vi "GenerateTdms.vi"   [LabVIEW 2011]
uses:
  <vilib>/Analysis/NI_AALBase.lvlib
types:
  T1 = enum16{"open", "open or create", "create or replace", "create", "open (read-only)"}
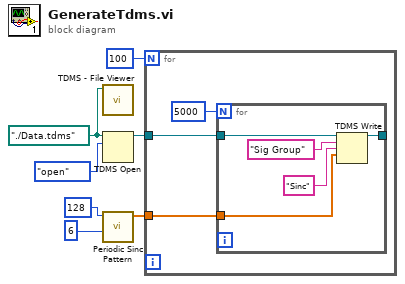
[diagram p0: block diagram]
diagram:
  w5 = path "./Data.tdms" ("文件路径")
  n1 = call <vilib>:"TDMS - File Viewer.vi"("file path"=w5) -> ()  [unwired: 5 in, 2 out]
  n2 = TDMS Open(10:T1."open" ("操作(0:open)"), 11:w5) -> (3:w6:refnum<k34>)  [unwired: 4 in, 1 out]
  n3 = call <vilib>:"Periodic Sinc Pattern.vi"("order"=6, "samples"=128) -> ("Periodic Sinc Pattern"=w2:dbl[])  [unwired: 8 in, 1 out]
  n4 = for {
    N: 100 -> [_]
    tunnel: w6 -> [w9]
    tunnel: w2 -> [w8]
    n5 = for {
      N: 5000 -> [_]
      tunnel: w9 -> [w15]
      tunnel: [w14] -> _
      tunnel: w8 -> [w12]
      n6 = TDMS Write(0:w15, 5:"Sig Group" ("组名称输入（无标题）"), 7:"Sinc", 9:w12) -> (4:w14:refnum<k34>)  [unwired: 2 in, 3 out]
    }
  }
